vi "ConvertEventEnum.vi"(3 "Button ID":T2(ring), 4 "Crtl1?":bool) -> (5 "4134 Button ID":T1(ring))   [LabVIEW 2010, in "FTC.lvlib" / "Remote Interface.lvlib"]
uses:
  Remote Interface.lvlib
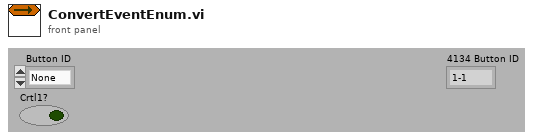
[diagram p1: front panel]
types:
  T1 = enum16{"1-1", "1-2", "1-3", "1-4", "1-5", "1-6", "1-7", "1-8", "1-9", "1-10", "1-11", "1-12", "2-1", "2-2", "2-3", "2-4", "2-5", "2-6", "2-7", "2-8", "2-9", "2-10", "2-11", "2-12", "NXT-L", "NXT-R", "NXT-E", "1-U", "1-UR", "1-R", "1-DR", "1-D", "1-DL", "1-L", "1-UL", "2-U", "2-UR", "2-R", "2-DR", "2-D", "2-DL", "2-L", "2-UL"}
  T2 = enum16{"None", "Button 1", "Button 2", "Button 3", "Button 4", "Button 5", "Button 6", "Button 7", "Button 8", "Button 9", "Button 10", "Button 11", "Button 12", "POV Up", "POV Up Right", "POV Right", "POV Down Right", "POV Down", "POV Down Left", "POV Left", "POV Up Left"}
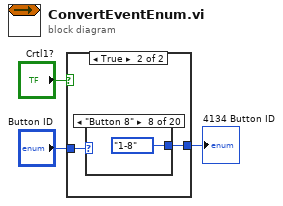
[diagram p0: block diagram]
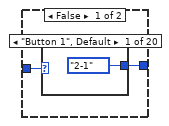
[diagram p2: hidden frame]
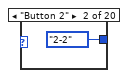
[diagram p3: hidden frame]
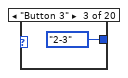
[diagram p4: hidden frame]
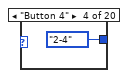
[diagram p5: hidden frame]
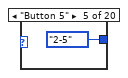
[diagram p6: hidden frame]
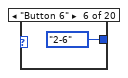
[diagram p7: hidden frame]
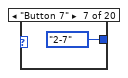
[diagram p8: hidden frame]
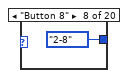
[diagram p9: hidden frame]
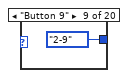
[diagram p10: hidden frame]
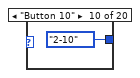
[diagram p11: hidden frame]
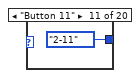
[diagram p12: hidden frame]
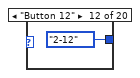
[diagram p13: hidden frame]
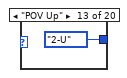
[diagram p14: hidden frame]
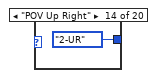
[diagram p15: hidden frame]
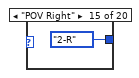
[diagram p16: hidden frame]
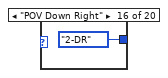
[diagram p17: hidden frame]
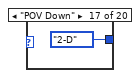
[diagram p18: hidden frame]
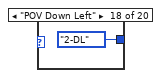
[diagram p19: hidden frame]
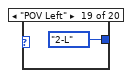
[diagram p20: hidden frame]
diagram:
  n1 = case shown="True" "Crtl1?" {
    tunnel: "Button ID" -> [w5 w27]
    tunnel: [w4 w26] -> w1
    frame False {
      n2 = case shown="\"Button 1\", Default" w5 {
        tunnel: [T1."2-1" ("4134 Button ID") T1."2-2" ("4134 Button ID") T1."2-3" ("4134 Button ID") T1."2-4" ("4134 Button ID") T1."2-5" ("4134 Button ID") T1."2-6" ("4134 Button ID") T1."2-7" ("4134 Button ID") T1."2-8" ("4134 Button ID") T1."2-9" ("4134 Button ID") T1."2-10" ("4134 Button ID") T1."2-11" ("4134 Button ID") T1."2-12" ("4134 Button ID") T1."2-U" ("4134 Button ID") T1."2-UR" ("4134 Button ID") T1."2-R" ("4134 Button ID") T1."2-DR" ("4134 Button ID") T1."2-D" ("4134 Button ID") T1."2-DL" ("4134 Button ID") T1."2-L" ("4134 Button ID") T1."2-UL" ("4134 Button ID")] -> w4
        frame "Button 1", Default {
        }
        frame "Button 2" {
        }
        frame "Button 3" {
        }
        frame "Button 4" {
        }
        frame "Button 5" {
        }
        frame "Button 6" {
        }
        frame "Button 7" {
        }
        frame "Button 8" {
        }
        frame "Button 9" {
        }
        frame "Button 10" {
        }
        frame "Button 11" {
        }
        frame "Button 12" {
        }
        frame "POV Up" {
        }
        frame "POV Up Right" {
        }
        frame "POV Right" {
        }
        frame "POV Down Right" {
        }
        frame "POV Down" {
        }
        frame "POV Down Left" {
        }
        frame "POV Left" {
        }
        frame "POV Up Left" {
        }
      }
    }
    frame True {
      n3 = case shown="\"Button 8\"" w27 {
        tunnel: [T1."1-1" ("4134 Button ID") T1."1-2" ("4134 Button ID") T1."1-3" ("4134 Button ID") T1."1-4" ("4134 Button ID") T1."1-5" ("4134 Button ID") T1."1-6" ("4134 Button ID") T1."1-7" ("4134 Button ID") T1."1-8" ("4134 Button ID") T1."1-9" ("4134 Button ID") T1."1-10" ("4134 Button ID") T1."1-11" ("4134 Button ID") T1."1-12" ("4134 Button ID") T1."1-U" ("4134 Button ID") T1."1-UR" ("4134 Button ID") T1."1-R" ("4134 Button ID") T1."1-DR" ("4134 Button ID") T1."1-D" ("4134 Button ID") T1."1-DL" ("4134 Button ID") T1."1-L" ("4134 Button ID") T1."1-UL" ("4134 Button ID")] -> w26
        frame "Button 1", Default {
        }
        frame "Button 2" {
        }
        frame "Button 3" {
        }
        frame "Button 4" {
        }
        frame "Button 5" {
        }
        frame "Button 6" {
        }
        frame "Button 7" {
        }
        frame "Button 8" {
        }
        frame "Button 9" {
        }
        frame "Button 10" {
        }
        frame "Button 11" {
        }
        frame "Button 12" {
        }
        frame "POV Up" {
        }
        frame "POV Up Right" {
        }
        frame "POV Right" {
        }
        frame "POV Down Right" {
        }
        frame "POV Down" {
        }
        frame "POV Down Left" {
        }
        frame "POV Left" {
        }
        frame "POV Up Left" {
        }
      }
    }
  }
  "4134 Button ID" <- w1
